vi "velocidade angular media.vi"(8 "Time Stamp 2":timestamp, 9 "tetha 2":dbl, 10 "Time Stamp 1":timestamp, 11 "tetha 1":dbl) -> (3 "angular speed (rad/s)":dbl)   [LabVIEW 2016]
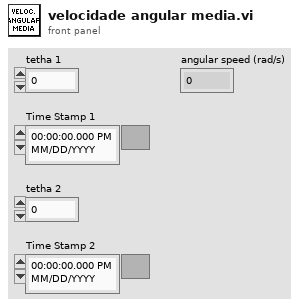
[diagram p1: front panel]
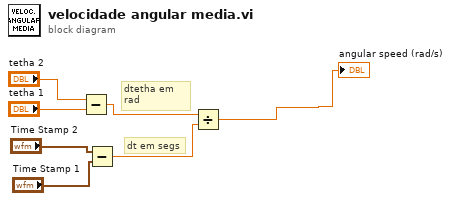
[diagram p0: block diagram]
diagram:
  # "dtetha em rad"
  # "dt em segs"
  n1 = Subtract(x="tetha 2", y="tetha 1") -> (x-y=w6:dbl)
  n2 = Subtract(x="Time Stamp 2", y="Time Stamp 1") -> (x-y=w7:dbl)
  n3 = Divide(x=w6, y=w7) -> (x/y=→"angular speed (rad/s)":dbl)
